vi "Quick Scale 1D PtByPt.vi"(0 "x":dbl format="%0.2f", 1 "sample length":i32=100, 2 "initialize":bool) -> (3 "Y[i]=X[i]/Max|X|":dbl[](array[numeric]), 4 "max|X|":dbl format="%0.2f", 5 "error":i32)   [LabVIEW 2020, in "NI_PtbyPt.lvlib"]
doc: "Determines the maximum absolute value contained in the set of input data points specified by <B>sample length</B> and then scales the set of input data points using the absolute value."
uses:
  <vilib>/ptbypt/NI_PtbyPt.lvlib
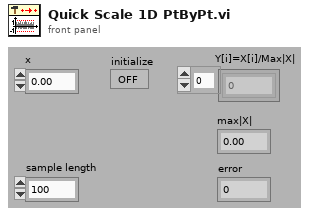
[diagram p1: front panel]
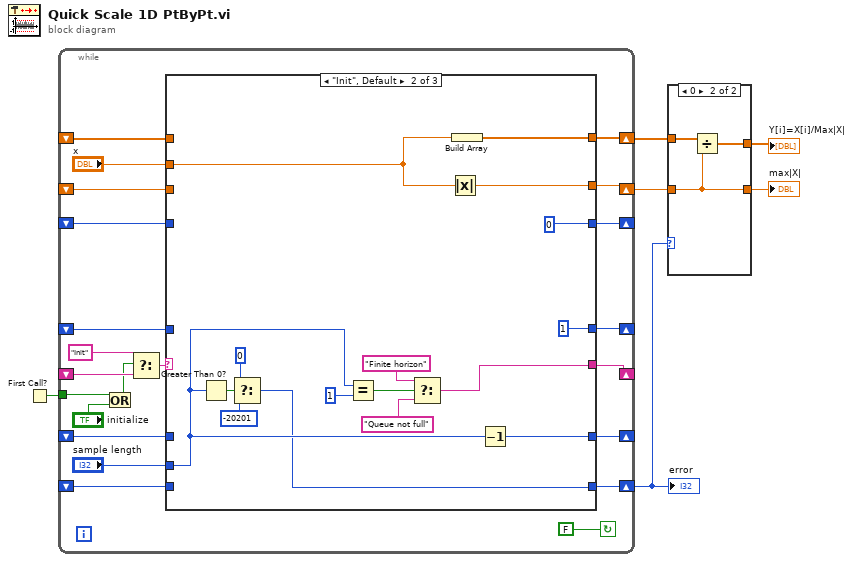
[diagram p0: block diagram]
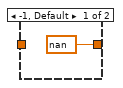
[diagram p2: hidden frame]
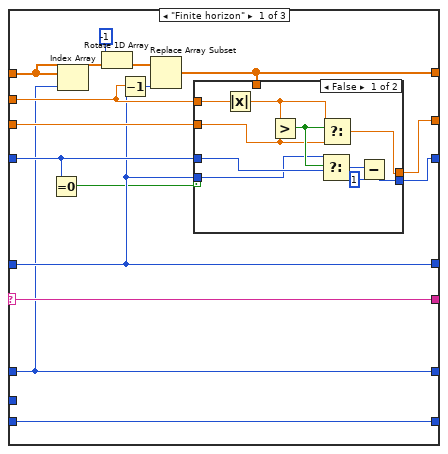
[diagram p3: hidden frame]
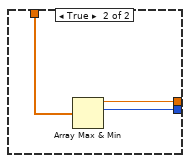
[diagram p4: hidden frame]
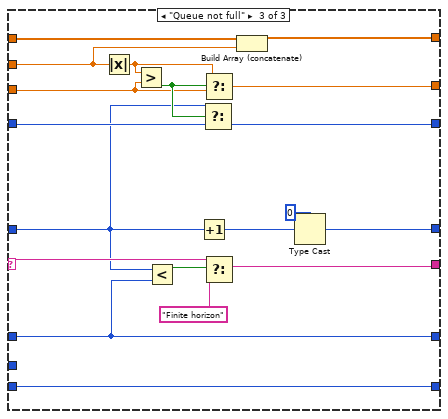
[diagram p5: hidden frame]
diagram:
  n1 = First Call?() -> (First Call?: T/F=w6:bool)
  n2 = while {
    shift-left: _ -> [w9]
    shift-right: [w10] -> _
    tunnel: w6 -> [w13]
    shift-left: _ -> [w17]
    shift-right: [w18] -> _
    shift-left: _ -> [w20]
    shift-right: [w19] -> w3
    shift-left: _ -> [w22]
    shift-right: [w21] -> w5
    shift-left: _ -> [w24]
    shift-right: [w25] -> _
    shift-left: _ -> [w28]
    shift-right: [w23] -> _
    shift-right: [w8] -> w1
    shift-left: _ -> [w7]
    stop <- FALSE continue-if-true
    n3 = Or(x=w13, y="initialize") -> (x .or. y?=w11:bool)
    n4 = Select(t="Init", s=w11, f=w28) -> (s? t:f=w26:string)
    n5 = case shown="\"Init\", Default" w26 {
      selector: w26 -> [w40 _ w85]
      tunnel: "x" -> [w36 w67 w75]
      tunnel: [w33 1 w88] -> w25
      tunnel: w24 -> [w33 _ w77]
      tunnel: [w40 w60 w83] -> w23
      tunnel: w22 -> [w38 _ w91]
      tunnel: [w37 w59 w90] -> w21
      tunnel: "sample length" -> [_ w62 _]
      tunnel: w20 -> [w35 _ w81]
      tunnel: [w39 w58 w78] -> w19
      tunnel: [w32 0 w79] -> w18
      tunnel: w17 -> [w34 _ w80]
      tunnel: [w31 w61 w76] -> w10
      tunnel: w9 -> [w31 _ w76]
      tunnel: [w29 w57 w73] -> w8
      tunnel: w7 -> [w29 _ w73]
      frame "Finite horizon" {
        n6 = Equal To 0?(x=w34) -> (x = 0?=w30:bool)
        n7 = Index Array(array=w38, index=w31) -> ()  [unwired: 1 out]
        n8 = Rotate 1D Array(1:w38, 2:i16 -1 ("n")) -> (0:w42:dbl[])
        n9 = Decrement(x=w33) -> (x-1=w41:i32)
        n10 = Replace Array Subset(array=w42, new element=w36, index=w41) -> (w37:dbl[])
        n11 = case shown="False" w30 {
          tunnel: w37 -> [_ w56]
          tunnel: [w49 w55] -> w39
          tunnel: [w46 w54] -> w32
          tunnel: w36 -> [w52 _]
          tunnel: w35 -> [w51 _]
          tunnel: w34 -> [w50 _]
          tunnel: w33 -> [w48 _]
          frame False {
            n12 = Absolute Value(x=w52) -> (abs(x)=w44:dbl)
            n13 = Greater?(x=w44, y=w51) -> (0:w53:bool)
            n14 = Select(t=w48, s=w53, f=w50) -> (s? t:f=w47:i32)
            n15 = Select(t=w44, s=w53, f=w51) -> (s? t:f=w49:dbl)
            n16 = Subtract(x=w47, y=1) -> (x-y=w46:i32)
          }
          frame True {
            n17 = Array Max & Min(array=w56) -> (max value=w55:dbl, max index (indices)=w54:i32)  [unwired: 2 out]
          }
        }
      }
      frame "Init", Default {
        n18 = Greater Than 0?(x=w62) -> (x > 0?=w65:bool)
        n19 = Select(t=0, s=w65, f=-20201) -> (s? t:f=w57:i32)
        n20 = Equal?(x=w62, y=1) -> (x = y?=w70:bool)
        n21 = Select(t="Finite horizon", s=w70, f="Queue not full") -> (s? t:f=w60:string)
        n22 = Absolute Value(x=w67) -> (abs(x)=w58:dbl)
        n23 = Build Array(w67) -> (w59:dbl[])
        n24 = Decrement(x=w62) -> (x-1=w61:i32)
      }
      frame "Queue not full" {
        n25 = Absolute Value(x=w75) -> (abs(x)=w74:dbl)
        n26 = Greater?(x=w74, y=w81) -> (0:w82:bool)
        n27 = Less?(x=w77, y=w76) -> (x < y?=w86:bool)
        n28 = Increment(x=w77) -> (x+1=w89:i32)
        n29 = Select(t=w77, s=w82, f=w80) -> (s? t:f=w79:i32)
        n30 = Select(t=w74, s=w82, f=w81) -> (s? t:f=w78:dbl)
        n31 = Select(t=w85, s=w86, f="Finite horizon") -> (s? t:f=w83:string)
        n32 = Build Array (concatenate)(w91, w75) -> (w90:dbl[])
        n33 = Type Cast(type=0, x=w89) -> (*(type *) &x=w88:i32)
      }
    }
  }
  "error" <- w1
  n34 = case shown="0" w1 {
    tunnel: w5 -> [_ w95]
    tunnel: [_ w94] -> w4
    tunnel: w3 -> [_ w93]
    tunnel: [nan w93] -> w2
    frame -1, Default {
    }
    frame 0 {
      n35 = Divide(x=w95, y=w93) -> (x/y=w94:dbl[])
    }
  }
  "Y[i]=X[i]/Max|X|" <- w4
  "max|X|" <- w2
